vi "系统报警板块.vi"() -> ()   [LabVIEW 2016, in "环境动力监测库.lvlib"]
uses:
  <vilib>/Utility/miscctls.llb/LVPointTypeDef.ctl
  <vilib>/ptbypt/NI_PtbyPt.lvlib
panel:
  out "湿度":string="75.5 %"
  out "室温":string="25.8 ℃"
  out "X6":bool caption="门禁开关_MJ"
  out "X5":bool caption="烟雾检测_YW"
  out "X4":bool caption="浸水检测_SJ"
  out "外部电源状态":u16(ring) caption="外部电源状态：" items=["正常", "异常"]
  out "当前报警状态":u16(ring) caption="当前报警状态：" items=["无报警"=0, "过压报警"=1, "欠压报警"=2, "过流报警"=4, "漏电报警"=8]
  out "通讯状态":u16(ring) caption="通讯状态：" items=["正常", "异常"]
  out "内部电源状态":u16(ring) caption="内部电源状态：" items=["异常", "正常"]
  # "系统报警板块"
  # "室温:"
  # "湿度:"
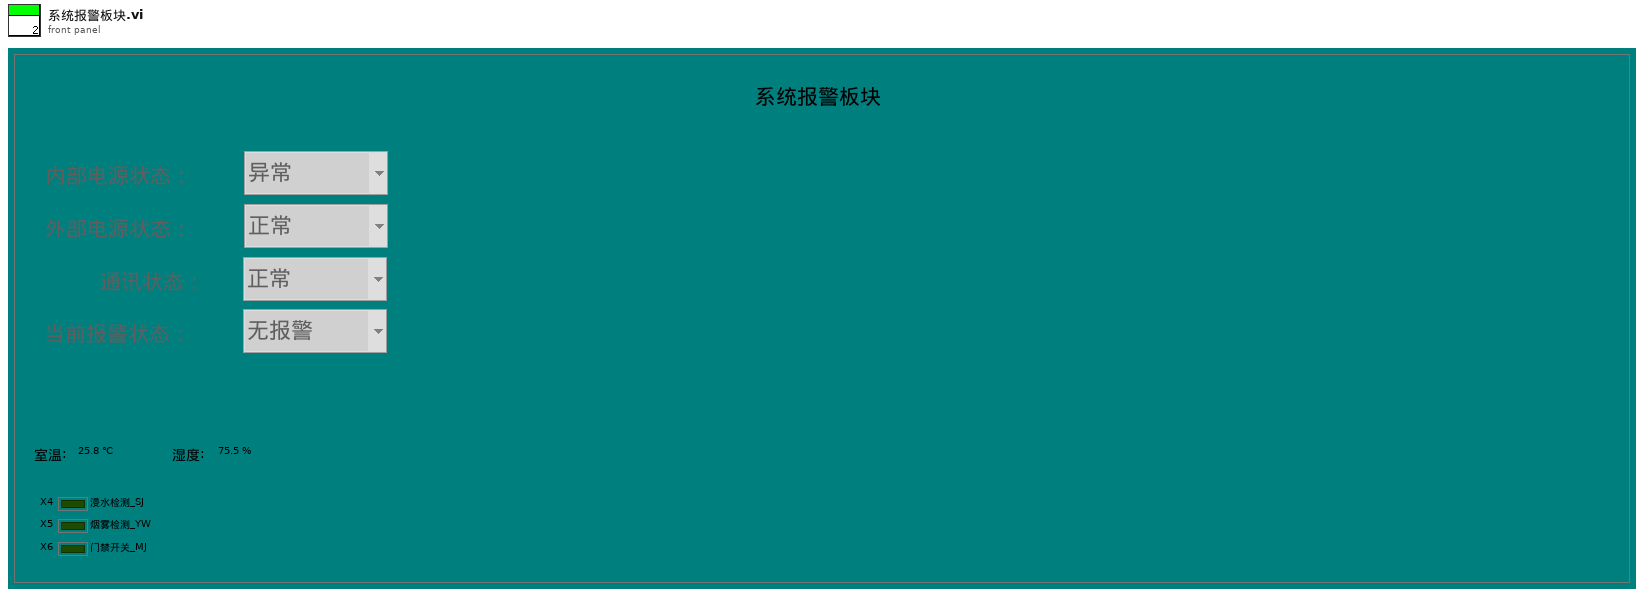
[diagram p1: front panel]
types:
  T1 = typedef "LVPointTypeDef.ctl" = cluster{"Horizontal":i16, "Vertical":i16}
  T2 = cluster{"AD0":sgl, "AD1":sgl, "AD2":sgl, "AD3":sgl, "AD4":sgl, "AD5":sgl}
  T3 = cluster{"R0":i16, "R1":i16, "R2":i16, "R3":i16, "R4":i16, "R5":i16, "R6":i16, "R7":i16, "R8":i16, "R9":i16, "R10":i16, "R11":i16, "R12":i16, "R13":i16, "R14":i16, "R15":i16, "R16":i16, "R17":i16, "R18":i16, "R19":i16, "R20":i16, "R21":i16, "R22":i16, "R23":i16, "R24":i16, "R25":i16, "R26":i16, "R27":i16, "R28":i16, "R29":i16, "R30":i16, "R31":i16, "R32":i16, "R33":i16, "R34":i16, "R35":i16, "R36":i16, "R37":i16, "R38":i16, "R39":i16}
  T4 = cluster{"时间标识":timestamp, "设备":string, "日志信息":string}
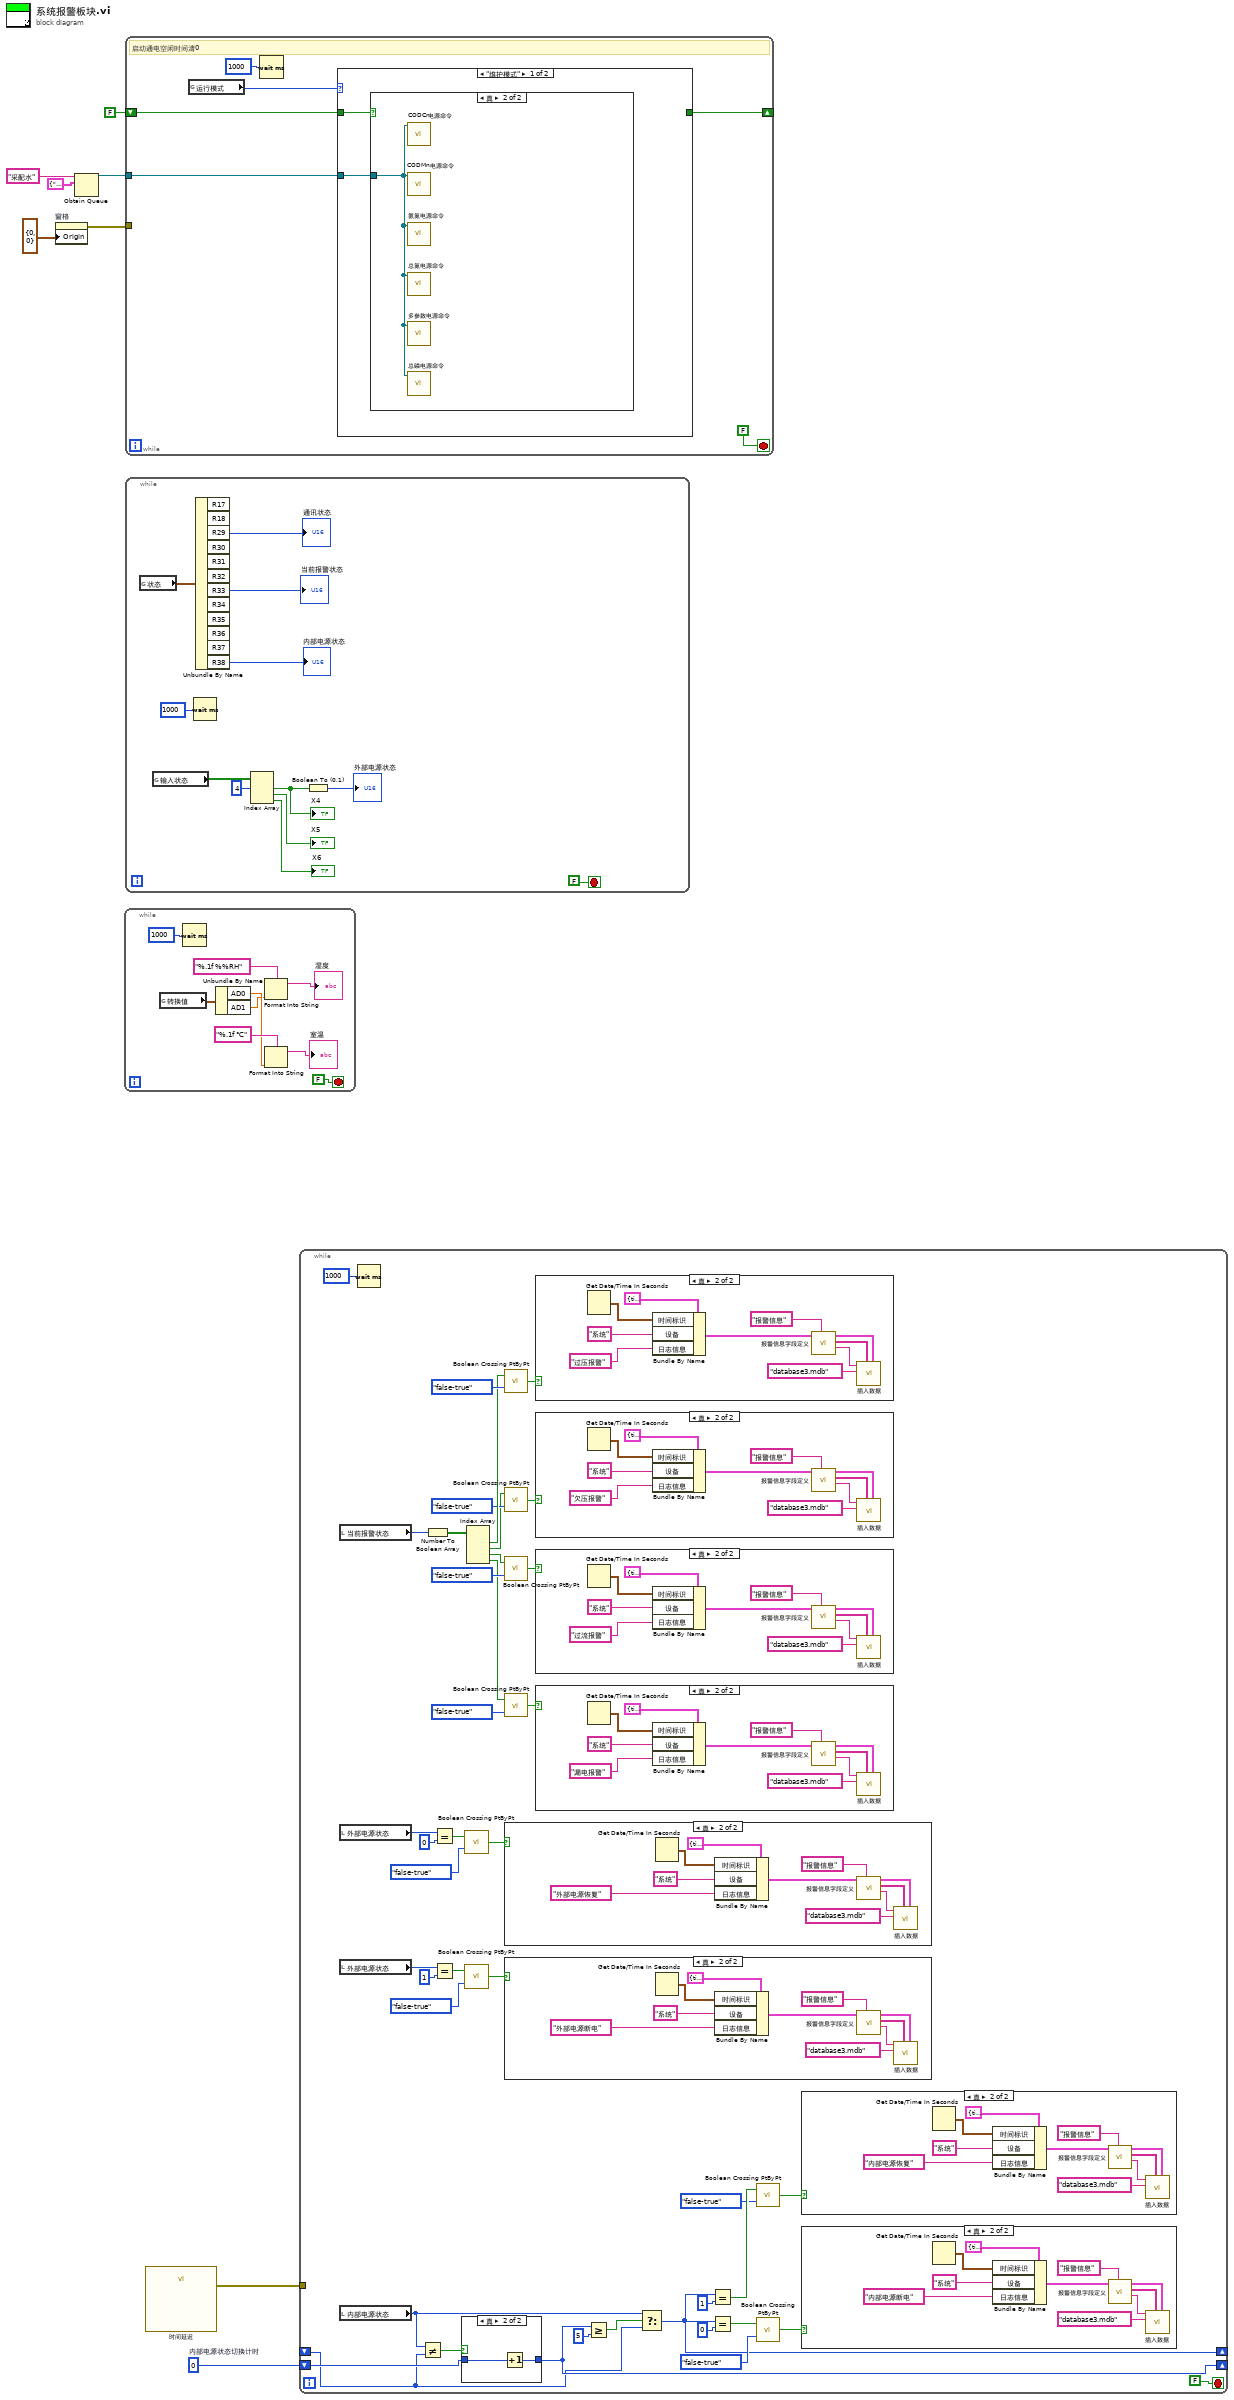
[diagram p0: block diagram]
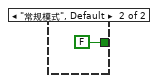
[diagram p12: hidden frame]
diagram:
  w2 = u16 0  # 内部电源状态切换计时
  n1 = property on="窗格" class="Pane"("Origin"=T1 {"Horizontal"=0, "Vertical"=0} ("原点")) -> (error out=w1:errorcluster)  [unwired: 2 in, 1 out]
  n2 = Obtain Queue(name (unnamed)="采配水" ("名称（未命名）"), element data type=cluster{"命令":string, "数据":variant} {"命令"="", "数据"=variant}) -> (queue out=w3:refnum<queue>)  [unwired: 3 in, 2 out]
  n3 = while {
    stop <- FALSE stop-if-true
    n4 = global read "外部交互全局变量.vi" "转换值"() -> (w11:T2)
    n5 = Wait (ms)(milliseconds to wait=u32 1000 ("等待时间（毫秒）")) -> ()  [unwired: 1 out]
    n6 = Unbundle By Name(w11) -> ("AD0"=w13:sgl, "AD1"=w12:sgl)
    n7 = Format Into String(format string="%.1f %%RH" ("格式字符串"), w12) -> (resulting string=→"湿度":string)  [unwired: 2 in, 1 out]
    n8 = Format Into String(format string="%.1f ℃" ("格式字符串"), w13) -> (resulting string=→"室温":string)  [unwired: 2 in, 1 out]
  }
  n9 = while {
    tunnel: w3 -> [w21]
    shift-right: [w19] -> _
    shift-left: FALSE -> [w20]
    tunnel: w1 -> [_]
    stop <- FALSE stop-if-true
    # "启动通电空闲时间清0"
    n10 = global read "外部交互全局变量.vi" "运行模式"() -> (w18:enum16{"维护模式", "常规模式", "应急模式", "质控模式"})
    n11 = Wait (ms)(milliseconds to wait=u32 1000 ("等待时间（毫秒）")) -> ()  [unwired: 1 out]
    n12 = case shown="\"维护模式\"" w18 {
      tunnel: w21 -> [w25 _]
      tunnel: w20 -> [w24 _]
      tunnel: [_ FALSE] -> w19
      frame "维护模式" {
        n13 = case shown="真" w24 {
          tunnel: w25 -> [_ w26]
          frame False {
          }
          frame True {
            n14 = call "CODCr电源命令.vi"("队列"=w26) -> ()  [unwired: 10 in, 1 out]
            n15 = call "CODMn电源命令.vi"("队列"=w26) -> ()  [unwired: 10 in, 1 out]
            n16 = call "氨氮电源命令.vi"("队列"=w26) -> ()  [unwired: 10 in, 1 out]
            n17 = call "总氮电源命令.vi"("队列"=w26) -> ()  [unwired: 10 in, 1 out]
            n18 = call "多参数电源命令.vi"("队列"=w26) -> ()  [unwired: 10 in, 1 out]
            n19 = call "总磷电源命令.vi"("队列"=w26) -> ()  [unwired: 10 in, 1 out]
          }
        }
      }
      frame "常规模式", Default {
      }
    }
  }
  n20 = while {
    stop <- FALSE stop-if-true
    n21 = global read "外部交互全局变量.vi" "状态"() -> (w32:T3)
    n22 = global read "外部交互全局变量.vi" "输入状态"() -> (w31:bool[])
    n23 = Wait (ms)(milliseconds to wait=u32 1000 ("等待时间（毫秒）")) -> ()  [unwired: 1 out]
    n24 = Unbundle By Name(w32) -> ("R29"=→"通讯状态":i16, "R33"=→"当前报警状态":i16, "R38"=→"内部电源状态":i16)  [unwired: 9 out]
    n25 = Index Array(array=w31, index #1=4 ("索引")) -> (element #1=w30:bool, element #2=→"X5":bool, element #3=→"X6":bool)  [unwired: 2 in]
    "X4" <- w30
    n26 = Boolean To (0,1)(Boolean=w30) -> (0, 1=→"外部电源状态":i16)
  }
  n27 = call "时间延迟"() -> ("error out"=w4:errorcluster)  [unwired: 11 in]
  n28 = while {
    tunnel: w4 -> [_]
    shift-right: [w45] -> _
    shift-left: w2 -> [w46]
    shift-right: [w40] -> _
    shift-left: _ -> [w41]
    stop <- FALSE stop-if-true
    n29 = local read "当前报警状态"() -> (w67:u16)
    n30 = local read "外部电源状态"() -> (w81:u16)
    n31 = local read "外部电源状态"() -> (w72:u16)
    n32 = local read "内部电源状态"() -> (w42:u16)
    n33 = Wait (ms)(milliseconds to wait=u32 1000 ("等待时间（毫秒）")) -> ()  [unwired: 1 out]
    n34 = Not Equal?(x=w42, y=w41) -> (x != y?=w51:bool)
    n35 = Number To Boolean Array(number=w67) -> (Boolean array=w66:bool[])
    n36 = Equal?(x=w81, y=u16 0) -> (x = y?=w79:bool)
    n37 = Equal?(x=w72, y=u16 1) -> (x = y?=w74:bool)
    n38 = case shown="真" w51 {
      tunnel: w46 -> [_ w93]
      tunnel: [_ w92] -> w45
      frame False {
      }
      frame True {
        n39 = Increment(x=w93) -> (x+1=w92:u16)
      }
    }
    n40 = call <vilib>:"Boolean Crossing PtByPt.vi"("direction"=enum16{"either", "false-true", "true-false"}."false-true", "input"=w79) -> ("crossing"=w77:bool)  [unwired: 1 in]
    n41 = call <vilib>:"Boolean Crossing PtByPt.vi"("direction"=enum16{"either", "false-true", "true-false"}."false-true", "input"=w74) -> ("crossing"=w76:bool)  [unwired: 1 in]
    n42 = Index Array(array=w66) -> (element #1=w64:bool, element #2=w58:bool, element #3=w57:bool, element #4=w54:bool)  [unwired: 4 in]
    n43 = call <vilib>:"Boolean Crossing PtByPt.vi"("direction"=enum16{"either", "false-true", "true-false"}."false-true", "input"=w64) -> ("crossing"=w63:bool)  [unwired: 1 in]
    n44 = call <vilib>:"Boolean Crossing PtByPt.vi"("direction"=enum16{"either", "false-true", "true-false"}."false-true", "input"=w58) -> ("crossing"=w62:bool)  [unwired: 1 in]
    n45 = call <vilib>:"Boolean Crossing PtByPt.vi"("direction"=enum16{"either", "false-true", "true-false"}."false-true", "input"=w57) -> ("crossing"=w59:bool)  [unwired: 1 in]
    n46 = call <vilib>:"Boolean Crossing PtByPt.vi"("direction"=enum16{"either", "false-true", "true-false"}."false-true", "input"=w54) -> ("crossing"=w56:bool)  [unwired: 1 in]
    n47 = case shown="真" w77 {
      frame False {
      }
      frame True {
        n48 = Get Date/Time In Seconds() -> (seconds since 1Jan1904=w162:timestamp)
        n49 = Bundle By Name(cluster=T4 {"时间标识"=timestamp(0 s since 1904-01-01), "设备"="", "日志信息"=""} ("data in"), "时间标识"=w162, "设备"="系统", "日志信息"="外部电源恢复") -> (w161:T4)
        n50 = call "报警信息字段定义.vi"("table输入"="报警信息", "data in"=w161) -> ("table输出"=w157:string, "columns"=w156:string[], "data out"=w155:T4)  [unwired: 7 in]
        n51 = call "插入数据.vi"("data"=w155, "columns"=w156, "database"="database3.mdb", "table"=w157) -> ()  [unwired: 7 in, 1 out]
      }
    }
    n52 = case shown="真" w76 {
      frame False {
      }
      frame True {
        n53 = Get Date/Time In Seconds() -> (seconds since 1Jan1904=w152:timestamp)
        n54 = Bundle By Name(cluster=T4 {"时间标识"=timestamp(0 s since 1904-01-01), "设备"="", "日志信息"=""} ("data in"), "时间标识"=w152, "设备"="系统", "日志信息"="外部电源断电") -> (w151:T4)
        n55 = call "报警信息字段定义.vi"("table输入"="报警信息", "data in"=w151) -> ("table输出"=w147:string, "columns"=w146:string[], "data out"=w145:T4)  [unwired: 7 in]
        n56 = call "插入数据.vi"("data"=w145, "columns"=w146, "database"="database3.mdb", "table"=w147) -> ()  [unwired: 7 in, 1 out]
      }
    }
    n57 = case shown="真" w63 {
      frame False {
      }
      frame True {
        n58 = Get Date/Time In Seconds() -> (seconds since 1Jan1904=w132:timestamp)
        n59 = Bundle By Name(cluster=T4 {"时间标识"=timestamp(0 s since 1904-01-01), "设备"="", "日志信息"=""} ("data in"), "时间标识"=w132, "设备"="系统", "日志信息"="过压报警") -> (w131:T4)
        n60 = call "报警信息字段定义.vi"("table输入"="报警信息", "data in"=w131) -> ("table输出"=w127:string, "columns"=w126:string[], "data out"=w125:T4)  [unwired: 7 in]
        n61 = call "插入数据.vi"("data"=w125, "columns"=w126, "database"="database3.mdb", "table"=w127) -> ()  [unwired: 7 in, 1 out]
      }
    }
    n62 = case shown="真" w62 {
      frame False {
      }
      frame True {
        n63 = Get Date/Time In Seconds() -> (seconds since 1Jan1904=w122:timestamp)
        n64 = Bundle By Name(cluster=T4 {"时间标识"=timestamp(0 s since 1904-01-01), "设备"="", "日志信息"=""} ("data in"), "时间标识"=w122, "设备"="系统", "日志信息"="欠压报警") -> (w121:T4)
        n65 = call "报警信息字段定义.vi"("table输入"="报警信息", "data in"=w121) -> ("table输出"=w117:string, "columns"=w116:string[], "data out"=w115:T4)  [unwired: 7 in]
        n66 = call "插入数据.vi"("data"=w115, "columns"=w116, "database"="database3.mdb", "table"=w117) -> ()  [unwired: 7 in, 1 out]
      }
    }
    n67 = case shown="真" w59 {
      frame False {
      }
      frame True {
        n68 = Get Date/Time In Seconds() -> (seconds since 1Jan1904=w112:timestamp)
        n69 = Bundle By Name(cluster=T4 {"时间标识"=timestamp(0 s since 1904-01-01), "设备"="", "日志信息"=""} ("data in"), "时间标识"=w112, "设备"="系统", "日志信息"="过流报警") -> (w111:T4)
        n70 = call "报警信息字段定义.vi"("table输入"="报警信息", "data in"=w111) -> ("table输出"=w107:string, "columns"=w106:string[], "data out"=w105:T4)  [unwired: 7 in]
        n71 = call "插入数据.vi"("data"=w105, "columns"=w106, "database"="database3.mdb", "table"=w107) -> ()  [unwired: 7 in, 1 out]
      }
    }
    n72 = case shown="真" w56 {
      frame False {
      }
      frame True {
        n73 = Get Date/Time In Seconds() -> (seconds since 1Jan1904=w102:timestamp)
        n74 = Bundle By Name(cluster=T4 {"时间标识"=timestamp(0 s since 1904-01-01), "设备"="", "日志信息"=""} ("data in"), "时间标识"=w102, "设备"="系统", "日志信息"="漏电报警") -> (w101:T4)
        n75 = call "报警信息字段定义.vi"("table输入"="报警信息", "data in"=w101) -> ("table输出"=w97:string, "columns"=w96:string[], "data out"=w95:T4)  [unwired: 7 in]
        n76 = call "插入数据.vi"("data"=w95, "columns"=w96, "database"="database3.mdb", "table"=w97) -> ()  [unwired: 7 in, 1 out]
      }
    }
    n77 = Greater Or Equal?(x=w45, y=u16 5) -> (x >= y?=w43:bool)
    n78 = Select(t=w42, s=w43, f=w41) -> (s? t:f=w40:u16)
    n79 = Equal?(x=w40, y=u16 1) -> (x = y?=w50:bool)
    n80 = Equal?(x=w40, y=u16 0) -> (x = y?=w69:bool)
    n81 = call <vilib>:"Boolean Crossing PtByPt.vi"("direction"=enum16{"either", "false-true", "true-false"}."false-true", "input"=w50) -> ("crossing"=w48:bool)  [unwired: 1 in]
    n82 = call <vilib>:"Boolean Crossing PtByPt.vi"("direction"=enum16{"either", "false-true", "true-false"}."false-true", "input"=w69) -> ("crossing"=w71:bool)  [unwired: 1 in]
    n83 = case shown="真" w48 {
      frame False {
      }
      frame True {
        n84 = Get Date/Time In Seconds() -> (seconds since 1Jan1904=w90:timestamp)
        n85 = Bundle By Name(cluster=T4 {"时间标识"=timestamp(0 s since 1904-01-01), "设备"="", "日志信息"=""} ("data in"), "时间标识"=w90, "设备"="系统", "日志信息"="内部电源恢复") -> (w89:T4)
        n86 = call "报警信息字段定义.vi"("table输入"="报警信息", "data in"=w89) -> ("table输出"=w85:string, "columns"=w84:string[], "data out"=w83:T4)  [unwired: 7 in]
        n87 = call "插入数据.vi"("data"=w83, "columns"=w84, "database"="database3.mdb", "table"=w85) -> ()  [unwired: 7 in, 1 out]
      }
    }
    n88 = case shown="真" w71 {
      frame False {
      }
      frame True {
        n89 = Get Date/Time In Seconds() -> (seconds since 1Jan1904=w142:timestamp)
        n90 = Bundle By Name(cluster=T4 {"时间标识"=timestamp(0 s since 1904-01-01), "设备"="", "日志信息"=""} ("data in"), "时间标识"=w142, "设备"="系统", "日志信息"="内部电源断电") -> (w141:T4)
        n91 = call "报警信息字段定义.vi"("table输入"="报警信息", "data in"=w141) -> ("table输出"=w137:string, "columns"=w136:string[], "data out"=w135:T4)  [unwired: 7 in]
        n92 = call "插入数据.vi"("data"=w135, "columns"=w136, "database"="database3.mdb", "table"=w137) -> ()  [unwired: 7 in, 1 out]
      }
    }
  }
